vi "SVM Train EPSILON_SVR.vi"(7 "Options":T9={"cache_size"=200.0, "eps"=0.001, "shrinking"=TRUE, "probability"=FALSE}, 8 "error in (no error)":errorcluster, 9 "Param EPSILON_SVR":T1={"C"=1.0, "p"=0.1}, 10 "Kernel":T8, 11 "Problem":T7) -> (0 "error out":errorcluster, 3 "Model":T2)   [LabVIEW 2014]
doc: "This function constructs and returns an SVM model according to the given training data and parameters."
uses:
  Controls/Options Training.ctl
  Controls/Kernel.ctl
  Wrapper API/Controls/svm_kernel_type.ctl
  Wrapper API/Controls/svm_problem.ctl
  Wrapper API/Controls/svm_node.ctl
  Wrapper API/Controls/svm_model.ctl
  Wrapper API/Controls/svm_parameter.ctl
  Wrapper API/Controls/svm_type.ctl
  Controls/Parameters EPSILON_SVR.ctl
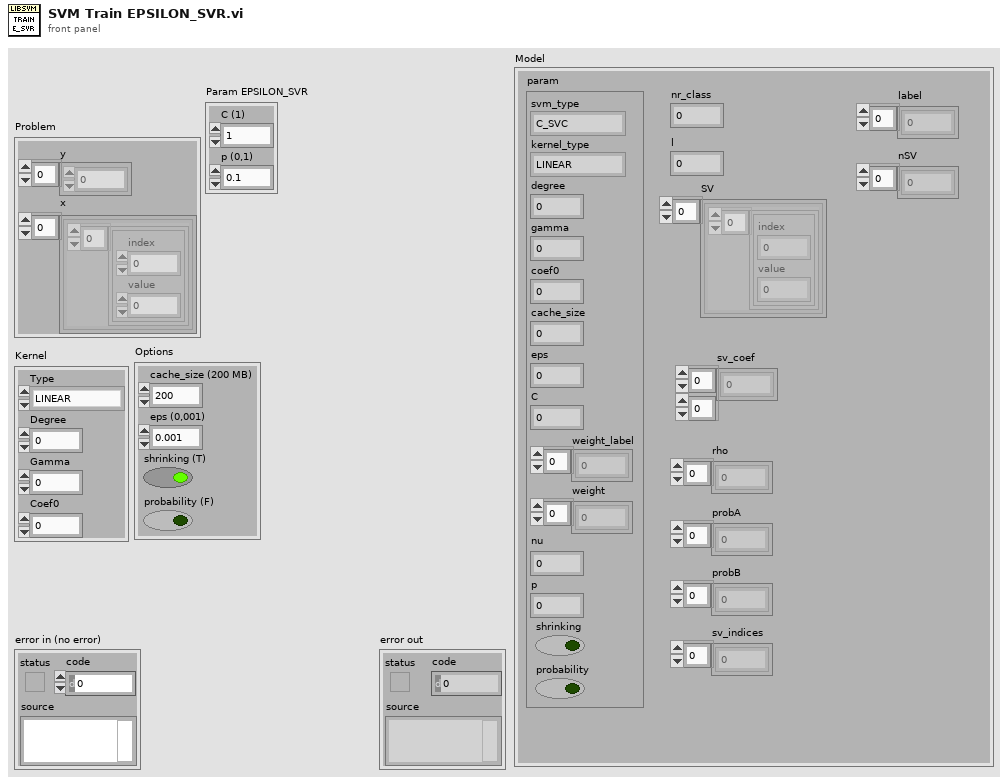
[diagram p1: front panel]
types:
  T1 = typedef "Parameters EPSILON_SVR.ctl" = cluster{"C":dbl, "p":dbl}
  T2 = typedef "svm_model.ctl" = cluster{"param":T3, "nr_class":i32, "l":i32, "SV":cluster{"Array":T6[]}[], "sv_coef":dbl[][], "rho":dbl[], "probA":dbl[], "probB":dbl[], "sv_indices":i32[], "label":i32[], "nSV":i32[]}
  T3 = typedef "svm_parameter.ctl" = cluster{"svm_type":T4, "kernel_type":T5, "degree":i32, "gamma":dbl, "coef0":dbl, "cache_size":dbl, "eps":dbl, "C":dbl, "weight_label":i32[], "weight":dbl[], "nu":dbl, "p":dbl, "shrinking":bool, "probability":bool}
  T4 = typedef "svm_type.ctl" = enum32{"C_SVC", "NU_SVC", "ONE_CLASS", "EPSILON_SVR", "NU_SVR"}
  T5 = typedef "svm_kernel_type.ctl" = enum32{"LINEAR", "POLY", "RBF", "SIGMOID", "PRECOMPUTED"}
  T6 = typedef "svm_node.ctl" = cluster{"index":i32, "value":dbl}
  T7 = typedef "svm_problem.ctl" = cluster{"y":dbl[], "x":cluster{T6[]}[]}
  T8 = typedef "Kernel.ctl" = cluster{"Type":T5, "Degree":i32, "Gamma":dbl, "Coef0":dbl}
  T9 = typedef "Options Training.ctl" = cluster{"cache_size":dbl, "eps":dbl, "shrinking":bool, "probability":bool}
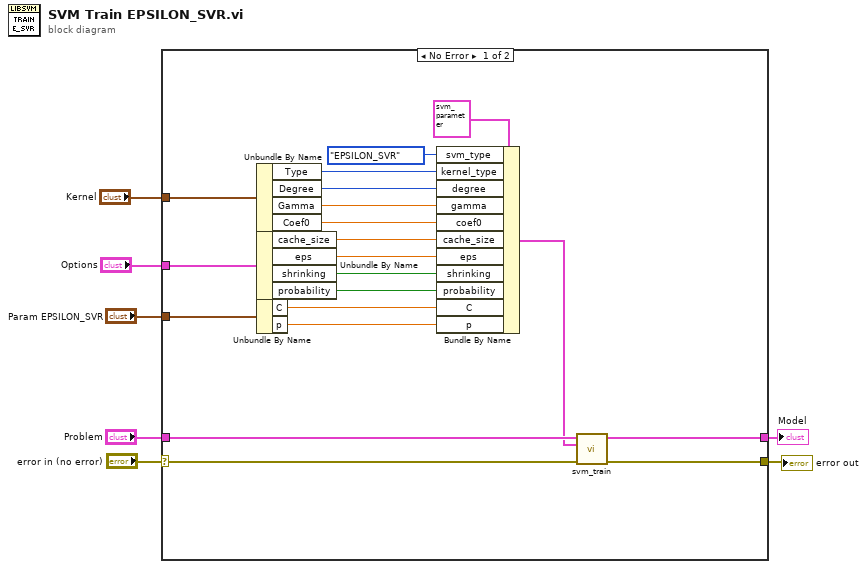
[diagram p0: block diagram]
diagram:
  n1 = case shown="No Error" "error in (no error)" {
    selector: "error in (no error)" -> [w27 w28]
    tunnel: [w26 w28] -> w7
    tunnel: "Problem" -> [w24 _]
    tunnel: "Kernel" -> [w23 _]
    tunnel: [w16 _] -> w3
    tunnel: "Options" -> [w12 _]
    tunnel: "Param EPSILON_SVR" -> [w13 _]
    frame No Error {
      n2 = Unbundle By Name(w23) -> ("Type"=w22:T5, "Degree"=w21:i32, "Gamma"=w20:dbl, "Coef0"=w19:dbl)
      n3 = Unbundle By Name(w12) -> ("cache_size"=w15:dbl, "eps"=w14:dbl, "shrinking"=w11:bool, "probability"=w10:bool)
      n4 = Unbundle By Name(w13) -> ("C"=w9:dbl, "p"=w8:dbl)
      n5 = Bundle By Name(cluster=T3 {"svm_type"=enum."C_SVC", "kernel_type"=enum."LINEAR", "degree"=0, "gamma"=0.0, "coef0"=0.0, "cache_size"=0.0, "eps"=0.0, "C"=0.0, "weight_label"=[], "weight"=[], "nu"=0.0, "p"=0.0, "shrinking"=FALSE, "probability"=FALSE} ("svm_parameter"), "svm_type"=svm_type."EPSILON_SVR", "kernel_type"=w22, "degree"=w21, "gamma"=w20, "coef0"=w19, "cache_size"=w15, "eps"=w14, "shrinking"=w11, "probability"=w10, "C"=w9, "p"=w8) -> (w17:T3)
      n6 = call "svm_train.vi"("error in (no error)"=w27, "Parameters"=w17, "Problem"=w24) -> ("error out"=w26:errorcluster, "Model"=w16:T2)  [unwired: 7 in]
    }
    frame Error {
    }
  }
  "error out" <- w7
  "Model" <- w3
